vi "CD Init_Prepare Async Data_BC to RT.vi"(8 "error in (no error)":errorcluster, 10 "Card Parameters (in)":T1, 11 "Channels In":T8[](array[typedef]) {"RTs"."Mode Codes"."Words Item Refs" format="%.0x"; "RTs"."Mode Codes"."Timestamp Channel Data Reference" format="%.0x"; "RTs"."subAddresses"."Words Item Refs" format="%.0x"; "RTs"."subAddresses"."Timestamp Channel Data Reference" format="%.0x"; "RTs"."Status Channel Data Reference" format="%.0x"; "RTs"."Command Channels Refs" format="%.0x"; "BC"."Acyclic Frames Trigger Channels Refs" format="%.0x"; "BC"."Command Channels Refs" format="%.0x"; "BC"."messages"."Timestamp Channel Data Reference" format="%.0x"; "BC"."messages"."Status Channel Data Refs" format="%.0x"; "BC"."messages"."Words Item Refs" format="%.0x"; "BC"."messages"."Words Block Data Refs"."Data Reference" format="%.0x"}) -> (0 "error out":errorcluster, 2 "Raw Values (BC to RT)":T3, 3 "Map (BC to RT)":T5[](array[typedef]) {"Channel Data Reference" format="%.0x"})   [LabVIEW 2017, in "Ballard MIL-1553 Engine.lvlib"]
doc: "This VI creates a static association between NI-VS FIFO Channel Index and Physical Channel, Label Index, Parameter Index for Parameter Channel of a Tx Scheduled Label."
uses:
  Ballard MIL-1553 Engine.lvlib
  Shared/Controls and Global/RT Channel.ctl
  Shared/Controls and Global/RT BC.ctl
  <vilib>/NI Veristand/Custom Device API/Custom Device Item Ref.ctl
  Shared/Controls and Global/RT Message.ctl
  Shared/Controls and Global/RT messageType.ctl
  Shared/Controls and Global/RT CWD1.ctl
  Shared/Controls and Global/RT CWD2.ctl
  <vilib>/NI Veristand/Custom Device API/Data Reference.ctl
  <vilib>/NI Veristand/Custom Device API/Block Data Reference.ctl
  Shared/Controls and Global/RT Remote Terminal.ctl
  Shared/Controls and Global/RT Remote Terminal_rtMode.ctl
  Shared/Controls and Global/RT Remote Terminal_RT subAddress.ctl
  Shared/Controls and Global/RT Remote Terminal_RT direction.ctl
  Shared/Controls and Global/RT Remote Terminal_RT Mode Code.ctl
  Controls/RT Async_Map BC2RT.ctl
  Controls/RT Async_Map_Type.ctl
  Controls/RT Async_Raw Values.ctl
  Controls/RT Async_Raw Values to Messages Index_Association.ctl
  Controls/Card Parameters.ctl
  Shared/Controls and Global/Initialization Method.ctl
  <vilib>/NI VeriStand/Custom Device API/Custom Device API.lvlib
  <instrlib>/BTI1553Lib/BTI1553LV.lvlib
  Shared/Ballard 1553 Shared.lvlib
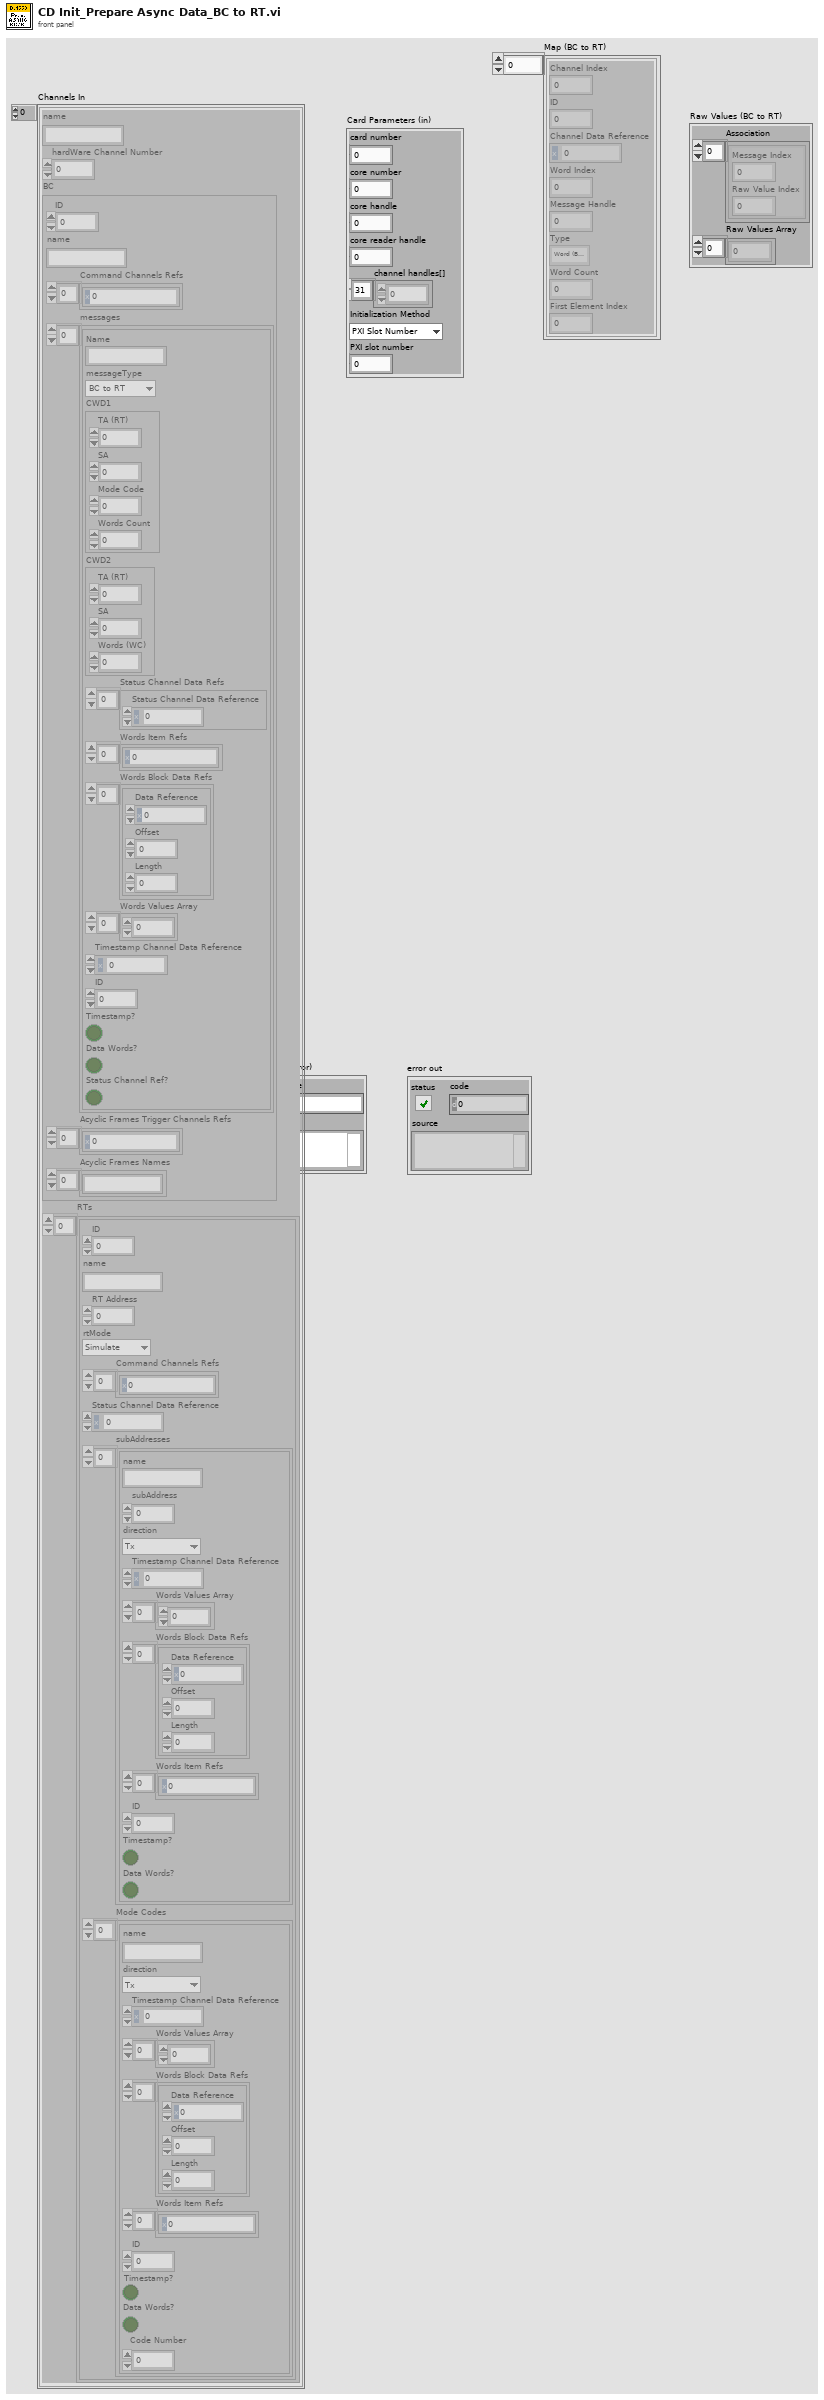
[diagram p1: front panel]
types:
  T1 = typedef "Ballard MIL-1553 Engine.lvlib/Card Parameters.ctl" = cluster{"card number":i32, "core number":i32, "core handle":u64, "core reader handle":u64, "channel handles[]":u64[], "Initialization Method":T2, "PXI slot number":i32}
  T2 = typedef "Ballard 1553 Shared.lvlib/Initialization Method.ctl" = enum16{"PXI Slot Number", "Card Number"}
  T3 = typedef "Ballard MIL-1553 Engine.lvlib/RT Async_Raw Values.ctl" = cluster{"Association":T4[], "Raw Values Array":u16[]}
  T4 = typedef "Ballard MIL-1553 Engine.lvlib/RT Async_Raw Values to Messages Index_Association.ctl" = cluster{"Message Index":i32, "Raw Value Index":i32}
  T5 = typedef "Ballard MIL-1553 Engine.lvlib/RT Async_Map BC2RT.ctl" = cluster{"Channel Index":i32, "ID":i32, "Channel Data Reference":T6, "Word Index":i32, "Message Handle":u64, "Type":T7, "Word Count":i32, "First Element Index":i32}
  T6 = typedef "Custom Device API.lvlib/Data Reference.ctl" = i32
  T7 = typedef "Ballard MIL-1553 Engine.lvlib/RT Async_Map_Type.ctl" = enum16{"Word (BC to RT)", "Word (MC (Rx))", "Acyclic Message Trigger", "Word (RT to ..)", "Word (RT to RT)", "Word (MC (Tx))", "RT Status", "BC Commands", "RT Commands"}
  T8 = typedef "Ballard 1553 Shared.lvlib/RT Channel.ctl" = cluster{"name":string, "hardWare Channel Number":u16, "BC":T9, "RTs":T16[]}
  T9 = typedef "Ballard 1553 Shared.lvlib/RT BC.ctl" = cluster{"ID":i32, "name":string, "Command Channels Refs":T10[], "messages":T11[], "Acyclic Frames Trigger Channels Refs":T10[], "Acyclic Frames Names":string[]}
  T10 = typedef "Custom Device API.lvlib/Custom Device Item Ref.ctl" = u64
  T11 = typedef "Ballard 1553 Shared.lvlib/RT Message.ctl" = cluster{"Name":string, "messageType":T12, "CWD1":T13, "CWD2":T14, "Status Channel Data Refs":T6[], "Words Item Refs":T10[], "Words Block Data Refs":T15[], "Words Values Array":u16[], "Timestamp Channel Data Reference":T6, "ID":i32, "Timestamp?":bool, "Data Words?":bool, "Status Channel Ref?":bool}
  T12 = typedef "Ballard 1553 Shared.lvlib/RT messageType.ctl" = enum16{"BC to RT", "RT to BC", "RT to RT", "MC (Rx)", "MC (Tx)"}
  T13 = typedef "Ballard 1553 Shared.lvlib/RT CWD1.ctl" = cluster{"TA (RT)":i8, "SA":i8, "Mode Code":i8, "Words Count":i8}
  T14 = typedef "Ballard 1553 Shared.lvlib/RT CWD2.ctl" = cluster{"TA (RT)":i8, "SA":i8, "Words (WC)":i8}
  T15 = typedef "Custom Device API.lvlib/Block Data Reference.ctl" = cluster{"Data Reference":T6, "Offset":u64, "Length":u64}
  T16 = typedef "Ballard 1553 Shared.lvlib/RT Remote Terminal.ctl" = cluster{"ID":i32, "name":string, "RT Address":i32, "rtMode":T17, "Command Channels Refs":T10[], "Status Channel Data Reference":T6, "subAddresses":T18[], "Mode Codes":T20[]}
  T17 = typedef "Ballard 1553 Shared.lvlib/RT Remote Terminal_rtMode.ctl" = enum16{"Simulate", "Monitor", "Disable"}
  T18 = typedef "Ballard 1553 Shared.lvlib/RT Remote Terminal_RT subAddress.ctl" = cluster{"name":string, "subAddress":i8, "direction":T19, "Timestamp Channel Data Reference":T6, "Words Values Array":u16[], "Words Block Data Refs":T15[], "Words Item Refs":T10[], "ID":i32, "Timestamp?":bool, "Data Words?":bool}
  T19 = typedef "Ballard 1553 Shared.lvlib/RT Remote Terminal_RT direction.ctl" = enum16{"Tx", "Rx"}
  T20 = typedef "Ballard 1553 Shared.lvlib/RT Remote Terminal_RT Mode Code.ctl" = cluster{"name":string, "direction":T19, "Timestamp Channel Data Reference":T6, "Words Values Array":u16[], "Words Block Data Refs":T15[], "Words Item Refs":T10[], "ID":i32, "Timestamp?":bool, "Data Words?":bool, "Code Number":i32}
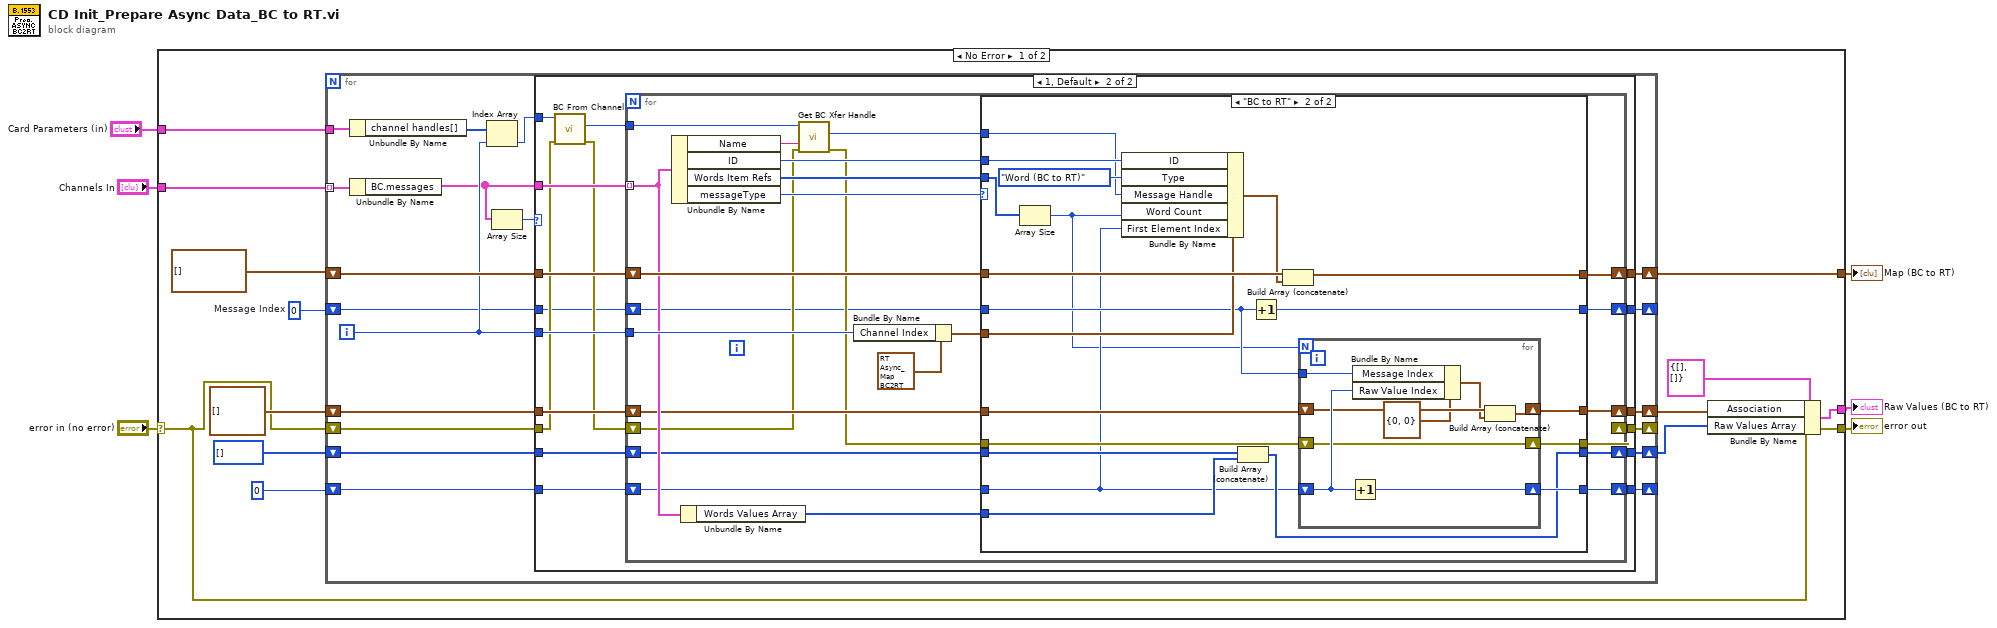
[diagram p0: block diagram]
diagram:
  n1 = case shown="No Error" "error in (no error)" {
    selector: "error in (no error)" -> [w9 w120]
    tunnel: [w9 w120] -> w5
    tunnel: "Channels In" -> [w19 _]
    tunnel: [w17 _] -> w3
    tunnel: [w13 _] -> w2
    tunnel: "Card Parameters (in)" -> [w10 _]
    frame No Error {
      w8 = 0  # Message Index
      n2 = for {
        tunnel: w19 -> [w38] mode=indexing
        shift-right: [w36] -> w17
        shift-left: T5[] [] -> [w37]
        shift-right: [w34] -> w14
        shift-left: T4[] [] -> [w35]
        shift-right: [w30] -> w7
        shift-left: u16[] [] -> [w33]
        shift-right: [w31] -> _
        shift-left: 0 -> [w32]
        tunnel: w10 -> [w29]
        shift-right: [w26] -> _
        shift-left: w9 -> [w24]
        shift-right: [w22] -> _
        shift-left: w8 -> [w23]
        i -> [w27]
        n3 = Unbundle By Name(w29) -> ("channel handles[]"=w28:u64[])
        n4 = Unbundle By Name(w38) -> ("BC.messages"=w20:T11[])
        n5 = Index Array(array=w28, index=w27) -> (element=w25:u64)
        n6 = Array Size(array=w20) -> (size(s)=w21:i32)
        n7 = case shown="1, Default" w21 {
          tunnel: w20 -> [_ w61]
          tunnel: w37 -> [w44 w60]
          tunnel: [w44 w59] -> w36
          tunnel: w35 -> [w42 w58]
          tunnel: [w42 w57] -> w34
          tunnel: w33 -> [w40 w56]
          tunnel: w32 -> [w39 w55]
          tunnel: [w39 w54] -> w31
          tunnel: [w40 w53] -> w30
          tunnel: w27 -> [_ w52]
          tunnel: [w41 w51] -> w26
          tunnel: w25 -> [_ w50]
          tunnel: w24 -> [w41 w49]
          tunnel: w23 -> [w43 w46]
          tunnel: [w43 w45] -> w22
          frame 0 {
          }
          frame 1, Default {
            n8 = call <instrlib>:"BC From Channel.vi"("error in (no error)"=w49, "channel handle in"=w50) -> ("error out"=w48:errorcluster, "bus controller handle out"=w47:u64)  [unwired: 7 in, 1 out]
            n9 = for {
              tunnel: w61 -> [w79] mode=indexing
              shift-right: [w64] -> w59
              shift-left: w60 -> [w83]
              tunnel: w52 -> [w84]
              shift-right: [w80] -> w57
              shift-left: w58 -> [w75]
              shift-right: [w78] -> w53
              shift-left: w56 -> [w74]
              shift-right: [w77] -> w54
              shift-left: w55 -> [w76]
              tunnel: w47 -> [w70]
              shift-right: [w66] -> w51
              shift-left: w48 -> [w68]
              shift-right: [w62] -> w45
              shift-left: w46 -> [w63]
              n10 = Unbundle By Name(w79) -> ("Name"=w69:string, "ID"=w71:i32, "Words Item Refs"=w81:T10[], "messageType"=w72:T12)
              n11 = Unbundle By Name(w79) -> ("Words Values Array"=w73:u16[])
              n12 = call <instrlib>:"Get BC Xfer Handle.vi"("error in (no error)"=w68, "bc transfer name"=w69, "bus controller handle in"=w70) -> ("error out"=w67:errorcluster, "bc transfer handle out"=w65:u64)  [unwired: 6 in, 1 out]
              n13 = Bundle By Name(cluster=T5 {"Channel Index"=0, "ID"=-1, "Channel Data Reference"=0, "Word Index"=0, "Message Handle"=0, "Type"=enum."Word (BC to RT)", "Word Count"=0, "First Element Index"=0} ("Association"), "Channel Index"=w84) -> (w82:T5)
              n14 = case shown="\"BC to RT\"" w72 {
                tunnel: w83 -> [w87 w100]
                tunnel: [w87 w99] -> w64
                tunnel: w82 -> [_ w97]
                tunnel: w81 -> [_ w94]
                tunnel: [w91 w111] -> w80
                tunnel: [w90 w106] -> w78
                tunnel: [w89 w110] -> w77
                tunnel: w76 -> [w89 w93]
                tunnel: w75 -> [w91 w109]
                tunnel: w74 -> [w90 w108]
                tunnel: w73 -> [_ w107]
                tunnel: w65 -> [_ w101]
                tunnel: w71 -> [_ w102]
                tunnel: w67 -> [w88 w105]
                tunnel: [w88 w104] -> w66
                tunnel: w63 -> [w86 w95]
                tunnel: [w86 w96] -> w62
                frame Default {
                  # "We don't care."
                }
                frame "BC to RT" {
                  n15 = Array Size(array=w94) -> (size(s)=w92:i32)
                  n16 = Bundle By Name(cluster=w97, "ID"=w102, "Type"=RT_Async_Map_Type."Word (BC to RT)", "Message Handle"=w101, "Word Count"=w92, "First Element Index"=w93) -> (w98:T5)
                  n17 = Build Array (concatenate)(w108, w107) -> (w106:u16[])
                  n18 = Increment(x=w95) -> (x+1=w96:i32)
                  n19 = Build Array (concatenate)(w100, w98) -> (w99:T5[])
                  n20 = for {
                    N: w92 -> [_]
                    shift-right: [w118] -> w110
                    shift-left: w93 -> [w117]
                    shift-right: [w115] -> w104
                    shift-left: w105 -> [w115]
                    tunnel: w95 -> [w112]
                    shift-right: [w119] -> w111
                    shift-left: w109 -> [w116]
                    n21 = Increment(x=w117) -> (x+1=w118:i32)
                    n22 = Bundle By Name(cluster=T4 {"Message Index"=0, "Raw Value Index"=0} ("Cluster"), "Message Index"=w112, "Raw Value Index"=w117) -> (w114:T4)
                    n23 = Build Array (concatenate)(w116, w114) -> (w119:T4[])
                  }
                }
              }
            }
          }
        }
      }
      n24 = Bundle By Name(cluster=T3 {"Association"=[], "Raw Values Array"=[]} ("Raw Values"), "Association"=w14, "Raw Values Array"=w7) -> (w13:T3)
    }
    frame Error {
    }
  }
  "error out" <- w5
  "Map (BC to RT)" <- w3
  "Raw Values (BC to RT)" <- w2
